vi "Create.vi"(6 "initial timestamp":timestamp, 8 "error in (no error)":errorcluster, 9 "choices":string[](array[string]), 10 "initial index":u16) -> (0 "error out":errorcluster, 1 "choices out":string[](array[string]), 2 "index out":u16, 3 "NT Enum out":refnum<class "NT Enum.lvclass">, 4 "timestamp out":timestamp)   [LabVIEW 2020, in "PV Access.lvlib" / "PV Data.lvlib" / "NT Enum.lvclass"]
uses:
  NT Enum.lvclass
  NT Enum.lvclass/NT Enum.ctl
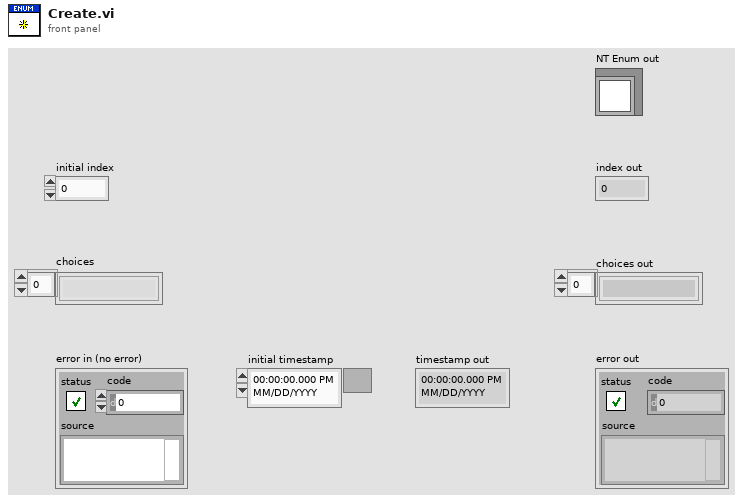
[diagram p1: front panel]
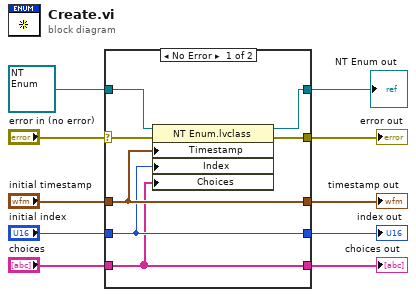
[diagram p0: block diagram]
diagram:
  n1 = case shown="No Error" "error in (no error)" {
    selector: "error in (no error)" -> [w17 w22]
    tunnel: [w14 w22] -> w9
    tunnel: [w15 w21] -> w7
    tunnel: refnum<class "NT Enum.lvclass"> refnum ("NT Enum in") -> [w16 w21]
    tunnel: "initial index" -> [w12 w19]
    tunnel: "choices" -> [w11 w18]
    tunnel: "initial timestamp" -> [w13 w20]
    tunnel: [w13 w20] -> w3
    tunnel: [w12 w19] -> w2
    tunnel: [w11 w18] -> w1
    frame No Error {
      n2 = property class="NT Enum.lvclass"(reference=w16, error in=w17, "Timestamp"=w13, "Index"=w12, "Choices"=w11) -> (reference out=w15:refnum<class "NT Enum.lvclass">, error out=w14:errorcluster)
    }
    frame Error {
    }
  }
  "error out" <- w9
  "NT Enum out" <- w7
  "timestamp out" <- w3
  "index out" <- w2
  "choices out" <- w1
